vi "temperaturemonitor.vi"() -> ()   [LabVIEW 2022 SP3]
panel:
  out "Warning":bool
  in  "High Limit":dbl
  out "Waveform Chart":cluster{dbl, "Thermometer":dbl}(graph)
  in  "Power":bool
  # "ON"
  # "OFF"
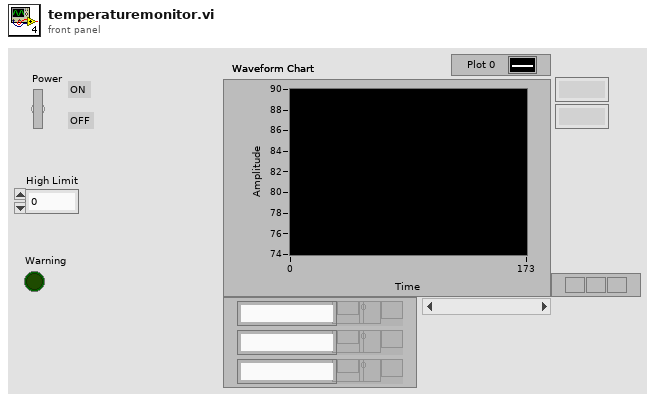
[diagram p1: front panel]
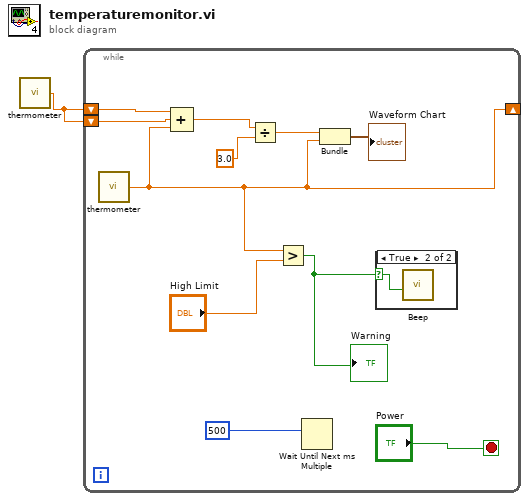
[diagram p0: block diagram]
diagram:
  n1 = call "thermometer.vi"() -> ("Thermometer"=w1:dbl)  [unwired: 1 in]
  n2 = while {
    shift-right: [w3] -> _
    shift-left: w1 -> [w10]
    shift-left: w1 -> [w9]
    stop <- "Power" stop-if-true
    n3 = call "thermometer.vi"() -> ("Thermometer"=w3:dbl)  [unwired: 1 in]
    n4 = Compound Arithmetic op=ADD(w10, w9, w3) -> (w12:dbl)
    n5 = Divide(x=w12, y=3.0) -> (x/y=w8:dbl)
    n6 = Greater?(x=w3, y="High Limit") -> (0:w2:bool)
    "Warning" <- w2
    n7 = Wait Until Next ms Multiple(millisecond multiple=500) -> ()  [unwired: 1 out]
    n8 = Bundle(w8, "Thermometer"=w3) -> (→"Waveform Chart":cluster{dbl, "Thermometer":dbl})  [unwired: 1 in]
    n9 = case shown="True" w2 {
      selector: w2 -> [_ w13]
      frame False {
      }
      frame True {
        n10 = call <vilib>:"Beep.vi"("use system alert? (T)"=w13) -> ()  [unwired: 11 in]
      }
    }
  }
